vi "hamamatsu_acquire.vi"(0 "Camera Acquire Settings":T1, 1 "# of images (in)":u32, 5 "last frame number acquired (in)":i32, 7 "ExperimentVariables (in)":refnum<class "ExperimentVariables.lvclass">, 11 "error in (no error)":errorcluster, 12 "Sum of Images (in)":u32[][](array[numeric])) -> (2 "# of images (out)":u32, 3 "ROI Pixel Count":u64[](array[numeric]), 4 "IMAQ Session Out":refnum<k11>, 6 "last frame number acquired (out)":i32, 8 "ExperimentVariables":refnum<class "ExperimentVariables.lvclass">, 10 "Image Array":T2[](array[plugin-control]), 14 "Sum of Images (out)":u32[][](array[numeric]), 15 "error out":errorcluster)   [LabVIEW 2013]
uses:
  ExperimentVariables/ExperimentVariables.lvclass
panel:
  out "ROI Array":u16[][](array[numeric])
  out "Image":T2(plugin-control)
  out "New Data?":bool
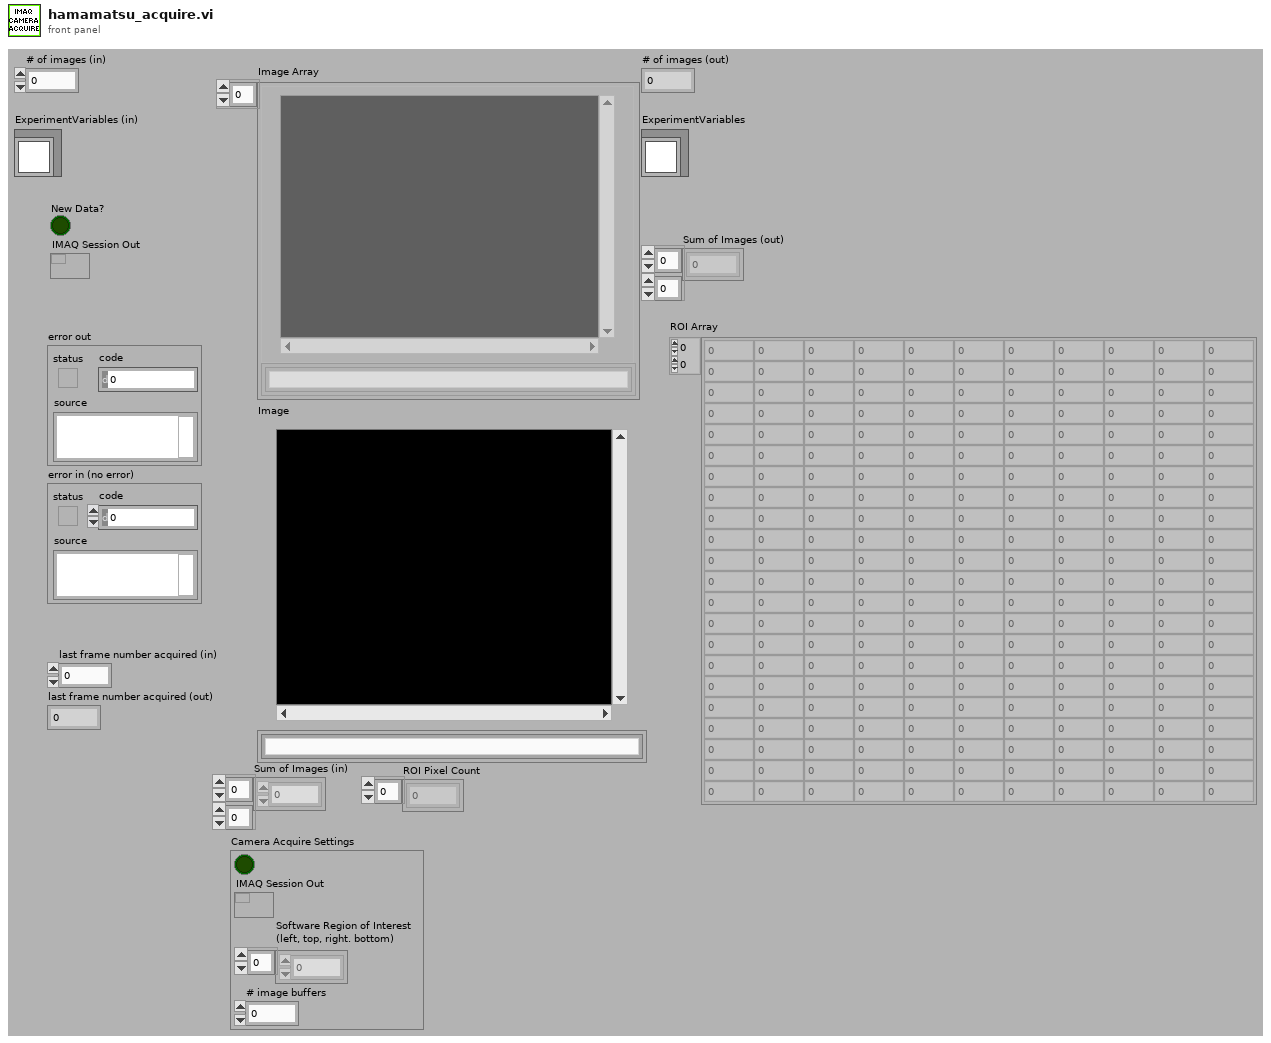
[diagram p1: front panel]
types:
  T1 = cluster{bool, "IMAQ Session Out":refnum<k11>, "Software Region of Interest\n(left, top, right. bottom)":i32[], "# image buffers":i32}
  T2 = typedef "IMAQ Image.ctl" = refnum<image>
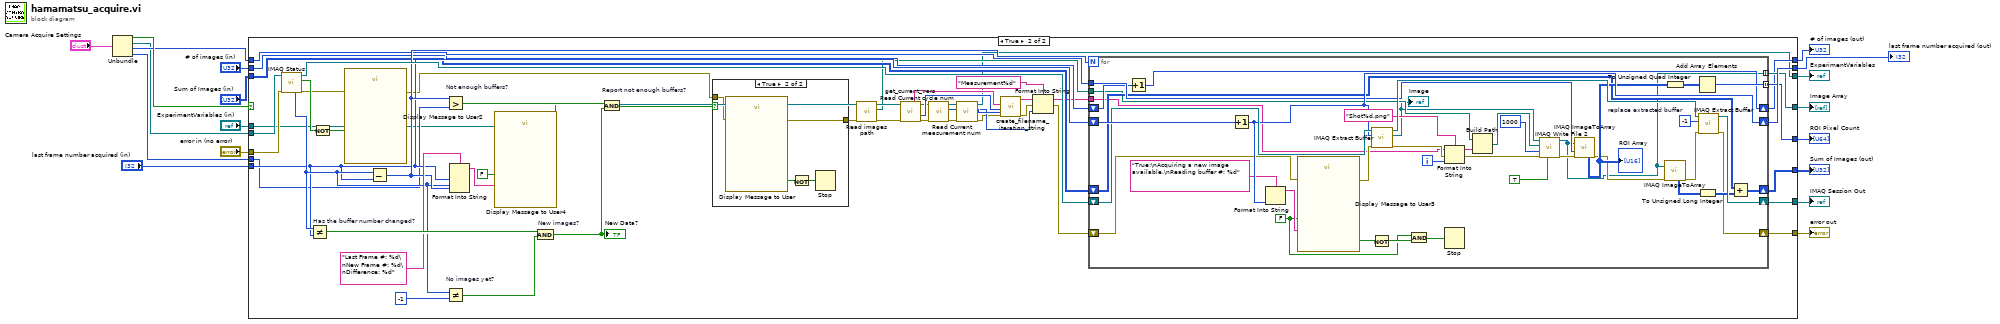
[diagram p0: block diagram]
diagram:
  n1 = Unbundle("Camera Acquire Settings") -> (w6:bool, "IMAQ Session Out"=w3:refnum<k11>, "Software Region of Interest\n(left, top, right. bottom)"=w4:i32[], "# image buffers"=w5:i32)
  n2 = case shown="True" w6 {
    tunnel: "error in (no error)" -> [w24 w59]
    tunnel: w4 -> [_ w58]
    tunnel: "last frame number acquired (in)" -> [w23 w57]
    tunnel: w5 -> [_ w56]
    tunnel: [w24 w55] -> w8
    tunnel: [w22 w54] -> w16
    tunnel: [w23 w53] -> w15
    tunnel: [_ w52] -> w14
    tunnel: [_ w51] -> w13
    tunnel: w3 -> [w22 w50]
    tunnel: [w21 w49] -> w12
    tunnel: "Sum of Images (in)" -> [w21 w48]
    tunnel: "# of images (in)" -> [w20 w47]
    tunnel: [w20 w46] -> w9
    tunnel: "ExperimentVariables (in)" -> [w19 w35]
    tunnel: [w19 w27] -> w1
    frame False {
    }
    frame True {
      n3 = call <vilib>:"IMAQ Status.vi"("error in (no error)"=w59, "IMAQ Session In"=w50) -> ("error out"=w65:errorcluster, "Acquiring?"=w67:bool, "IMAQ Session Out"=w73:refnum<k11>, "Last Valid Buffer Number"=w62:i32)  [unwired: 5 in, 1 out]
      n4 = Not Equal? "Has the buffer number changed?"(x=w62, y=w57) -> (x != y?=w69:bool)
      n5 = Not(x=w67) -> (.not. x?=w66:bool)
      n6 = call "Display Message to User2"("error in (no error)"=w65, "Enable"=w66) -> ("error out"=w45:errorcluster)  [unwired: 8 in, 1 out]
      n7 = Subtract(x=w62, y=w57) -> (x-y=w63:i32)
      n8 = Greater? "Not enough buffers?"(x=w63, y=w56) -> (0:w71:bool)
      n9 = Not Equal? "No images yet?"(x=w62, y=-1) -> (x != y?=w68:bool)
      n10 = Format Into String(format string="Last Frame #: %d\nNew Frame #: %d\nDifference: %d", w57, w62, w63) -> (resulting string=w61:string)  [unwired: 2 in, 1 out]
      n11 = call "Display Message to User4"("Enable"=FALSE, "Message"=w61) -> ()  [unwired: 8 in, 2 out]
      n12 = Compound Arithmetic op=AND "New images?"(w69, w68) -> (w74:bool)
      "New Data?" <- w74
      n13 = And "Report not enough buffers?"(x=w71, y=w74) -> (x .and. y?=w70:bool)
      n14 = case shown="True" w70 {
        tunnel: w45 -> [w115 w117]
        tunnel: [w115 w116] -> w37
        frame False {
        }
        frame True {
          n15 = call "Display Message to User"("error in (no error)"=w117) -> ("error out"=w116:errorcluster, "OK"=w118:bool)  [unwired: 9 in]
          n16 = Not(x=w118) -> (.not. x?=w119:bool)
          n17 = Stop(stop? (T)=w119) -> ()
        }
      }
      n18 = call-dynamic "Read images path.vi"("error in (no error)"=w37, "ExperimentVariables in"=w35) -> ("error out"=w36:errorcluster, "images path"=w33:path, "ExperimentVariables out"=w34:refnum<class "ExperimentVariables.lvclass">)  [unwired: 7 in]
      n19 = call-dynamic "get_current_vars.vi"("error in (no error)"=w36, "ExperimentVariables in"=w34) -> ("error out"=w30:errorcluster, "current variable indicies"=w43:i32[], "ExperimentVariables out"=w31:refnum<class "ExperimentVariables.lvclass">, "variable names"=w44:string[])  [unwired: 4 in, 2 out]
      n20 = call-dynamic "Read Current cycle num.vi"("error in (no error)"=w30, "ExperimentVariables in"=w31) -> ("error out"=w26:errorcluster, "Current cycle #"=w32:i32, "ExperimentVariables out"=w28:refnum<class "ExperimentVariables.lvclass">)  [unwired: 7 in]
      n21 = call-dynamic "Read Current measurement num.vi"("error in (no error)"=w26, "ExperimentVariables in"=w28) -> ("error out"=w25:errorcluster, "Current measurement #"=w29:i32, "ExperimentVariables out"=w27:refnum<class "ExperimentVariables.lvclass">)  [unwired: 7 in]
      n22 = call "create_filename_iteration_string.vi"(6:w32, "error in (no error)"=w25, "variable indices"=w43, "Variable Names Array"=w44) -> ("error out"=w40:errorcluster, "XYZ iteration string"=w42:string)  [unwired: 6 in]
      n23 = Format Into String(format string="Measurement%d", initial string=w42, error in=w40, w29) -> (resulting string=w38:string, error out=w39:errorcluster)
      n24 = for {
        N: w63 -> [_]
        shift-right: [w111] -> w53
        shift-left: w57 -> [w114]
        shift-right: [w106] -> w54
        shift-left: w73 -> [w113]
        shift-right: [w88] -> w55
        shift-left: w39 -> [w101]
        tunnel: [w77] -> w51 mode=indexing
        tunnel: [w102] -> w52 mode=indexing
        tunnel: w58 -> [w99]
        shift-right: [w96] -> w49
        shift-left: w48 -> [w95]
        shift-right: [w92] -> w46
        shift-left: w47 -> [w93]
        tunnel: w33 -> [w80]
        tunnel: w38 -> [w84]
        i -> [w82]
        w104 = FALSE ("Enable")
        w108 = -1  # replace extracted buffer
        n25 = Increment(x=w93) -> (x+1=w92:u32)
        n26 = Increment(x=w114) -> (x+1=w111:i32)
        n27 = Format Into String(format string="True:\nAcquiring a new image available.\nReading buffer #: %d", w111) -> (resulting string=w109:string)  [unwired: 2 in, 1 out]
        n28 = call "Display Message to User3"("error in (no error)"=w101, "Enable"=w104, "Message"=w109) -> ("error out"=w90:errorcluster, "OK"=w112:bool)  [unwired: 7 in]
        n29 = Not(x=w112) -> (.not. x?=w105:bool)
        n30 = call <vilib>:"IMAQ Extract Buffer.vi"("error in (no error)"=w90, "Buffer to extract"=w111, "IMAQ Session In"=w113) -> ("error out"=w86:errorcluster, "Image Out"=w78:T2, "IMAQ Session Out"=w107:refnum<k11>)  [unwired: 3 in, 3 out]
        "Image" <- w78
        n31 = And(x=w104, y=w105) -> (x .and. y?=w103:bool)
        n32 = Format Into String(format string="Shot%d.png", initial string=w84, error in=w86, w82) -> (resulting string=w81:string, error out=w85:errorcluster)
        n33 = Stop(stop? (T)=w103) -> ()
        n34 = Build Path(base path=w80, name or relative path=w81) -> (appended path=w79:path)
        n35 = call-poly "IMAQ Write File 2"("Use bit depth? (false)"=TRUE, "error in (no error)"=w85, "Image Quality"=u32 1000, "File Path"=w79, "Image"=w78) -> ("error out"=w87:errorcluster, "Image Out (duplicate)"=w77:T2)  [unwired: 5 in]
        n36 = call "IMAQ ImageToArray"("error in (no error)"=w87, "Optional Rectangle"=w99, "Image"=w77) -> ("Image Pixels (U16)"=w98:u16[][], "error out"=w91:errorcluster)  [unwired: 1 in, 3 out]
        "ROI Array" <- w98
        n37 = To Unsigned Quad Integer(1:w98) -> (0:w100:u64[][])
        n38 = call "IMAQ ImageToArray"("error in (no error)"=w91, "Image"=w77) -> ("Image Pixels (U16)"=w97:u16[][], "error out"=w89:errorcluster)  [unwired: 2 in, 3 out]
        n39 = Add Array Elements(numeric array=w100) -> (sum=w102:u64)
        n40 = To Unsigned Long Integer(number=w97) -> (unsigned 32bit integer=w94:u32[][])
        n41 = call <vilib>:"IMAQ Extract Buffer.vi"("error in (no error)"=w89, "Buffer to extract"=w108, "IMAQ Session In"=w107) -> ("error out"=w88:errorcluster, "IMAQ Session Out"=w106:refnum<k11>)  [unwired: 3 in, 4 out]
        n42 = Add(x=w95, y=w94) -> (x+y=w96:u32[][])
      }
    }
  }
  "error out" <- w8
  "IMAQ Session Out" <- w16
  "last frame number acquired (out)" <- w15
  "ROI Pixel Count" <- w14
  "Image Array" <- w13
  "Sum of Images (out)" <- w12
  "# of images (out)" <- w9
  "ExperimentVariables" <- w1
